vi "Ophir_ACQ.vi"(8 "error in (no error)":errorcluster, 10 "Background":dbl, 11 "Instruments in":refnum<class "Instruments.lvclass">) -> (0 "error out":errorcluster, 1 "Remeasure?":bool, 2 "Power,uW":dbl, 3 "Instruments out":refnum<class "Instruments.lvclass">, 5 "Back":dbl format="%0.2f")   [LabVIEW 2012, in "Instruments.lvclass"]
uses:
  Instruments.lvclass
  Instruments.lvclass/Instruments.ctl
  <vilib>/Analysis/NI_AALBase.lvlib
panel:
  out "Ophir_Param.Calibration Wl":dbl
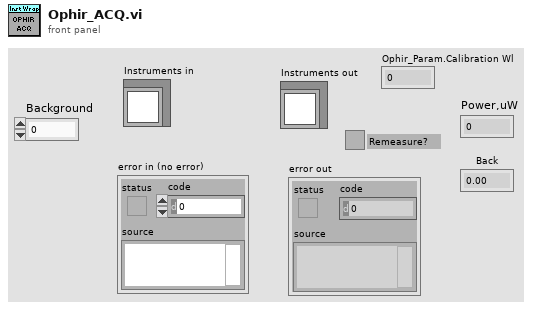
[diagram p1: front panel]
types:
  T1 = typedef "USB4000_Data.ctl" = cluster{"Wrapper Out":u32, "Number of Spectrometers":i32, "Wavelength":dbl[], "EL Spectrum":dbl[], "Int Time (usec)":i32, bool, "Background":dbl[]}
  T2 = cluster{"Keithley_Param":cluster{"Start Current,mA":dbl, "Stop Current,mA":dbl, "Voltage Compliance,V":dbl, "GPIB":string}, "USB4000_Param":cluster{"Integration Time":i32, "Wl min,nm":dbl, "Wl max,nm":dbl, "USB4000":T1}, "Ophir_Param":cluster{"VISA resource name":refnum<visa-resource-name>, "Calibration Wl":dbl}}
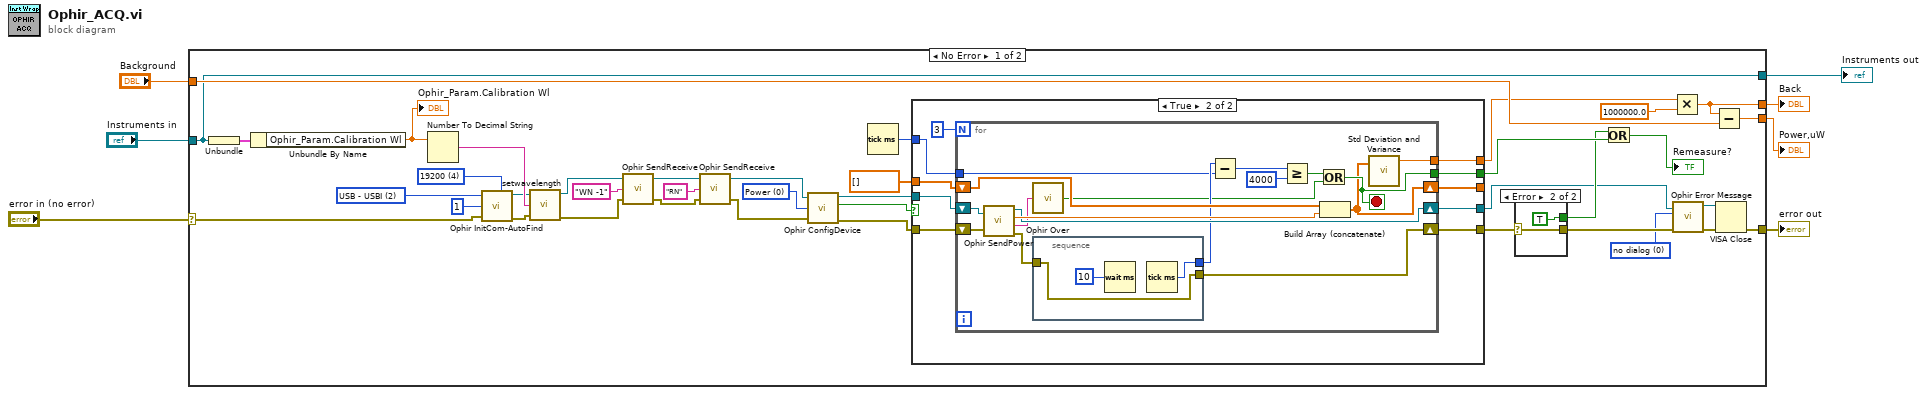
[diagram p0: block diagram]
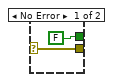
[diagram p2: hidden frame]
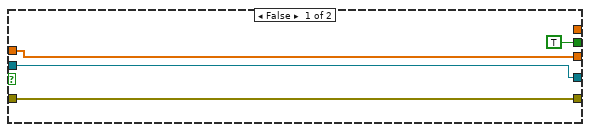
[diagram p3: hidden frame]
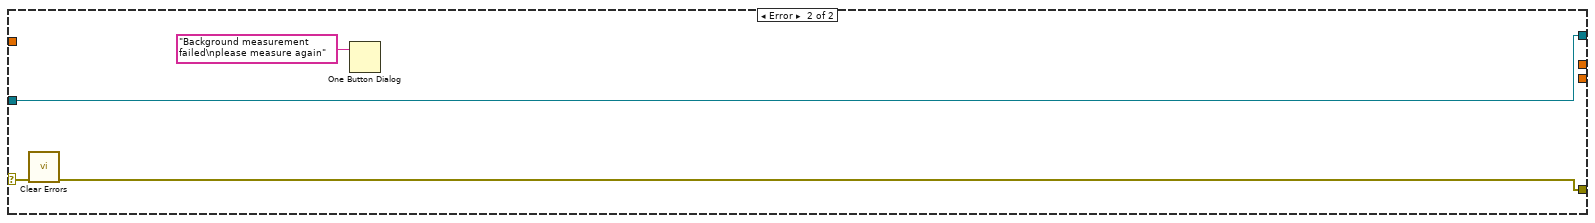
[diagram p4: hidden frame]
diagram:
  n1 = case shown="No Error" "error in (no error)" {
    selector: "error in (no error)" -> [w17 w86]
    tunnel: [w12 w85] -> w6
    tunnel: [w9 w88] -> w4
    tunnel: "Instruments in" -> [w9 w88]
    tunnel: "Background" -> [w24 _]
    tunnel: [w25 _] -> w2
    tunnel: [w23 _] -> w1
    frame No Error {
      w8 = 0 items=["no dialog", "OK message", "continue or stop message"] ("Type of Dialog (OK msg:1)")
      w18 = i16 4 items=["300", "1200", "4800", "9600", "19200", "38400"] ("Baud Rate (3:9600)")
      w20 = i16 2 items=["USB - Nova2", "USB - Vega", "USB - USBI", "RS232", "GPIB"] ("communication")
      w41 = u16 0 items=["Power", "Energy", "Frequency"] ("Measure Choice (0:Power)")
      n2 = Unbundle(w9) -> (w32:T2)
      n3 = Unbundle By Name(w32) -> ("Ophir_Param.Calibration Wl"=w21:dbl)
      "Ophir_Param.Calibration Wl" <- w21
      n4 = Number To Decimal String(number=w21) -> (decimal integer string=w33:string)  [unwired: 1 in]
      n5 = call "Ophir InitCom-AutoFind.vi"("Baud Rate (3:9600)"=w18, "communication"=w20, "Port Number (default 2)"=i16 1, "error in (no error)"=w17) -> ("Dup Visa Session"=w15:refnum<visa-resource-name>, "error out"=w16:errorcluster)  [unwired: 2 out]
      n6 = call "setwavelength.vi"("Dup Visa Session"=w15, "Set Wavelength"=w33, "error in (no error)"=w16) -> ("dup Visa Session"=w45:refnum<visa-resource-name>, "error out"=w44:errorcluster)  [unwired: 3 in]
      n7 = call "Ophir SendReceive.vi"("error in (no error)"=w44, "Command"="WN -1", "Visa Session"=w45) -> ("error out"=w29:errorcluster, "dup Visa Session"=w43:refnum<visa-resource-name>)  [unwired: 1 out]
      n8 = call "Ophir SendReceive.vi"("error in (no error)"=w29, "Command"="RN", "Visa Session"=w43) -> ("error out"=w39:errorcluster, "dup Visa Session"=w40:refnum<visa-resource-name>)  [unwired: 1 out]
      n9 = call "Ophir ConfigDevice.vi"("Visa Session"=w40, "Measure Choice (0:Power)"=w41, "error in (no error)"=w39) -> ("dup Visa Session"=w36:refnum<visa-resource-name>, "OK ?"=w38:bool, "error out"=w37:errorcluster)  [unwired: 1 out]
      n10 = Tick Count (ms)() -> (millisecond timer value=w30:u32)
      n11 = case shown="True" w38 {
        tunnel: w37 -> [w53 w62]
        tunnel: w36 -> [w54 w63]
        tunnel: dbl[] [] -> [w52 w64]
        tunnel: [w54 w61] -> w10
        tunnel: [w53 w60] -> w31
        tunnel: [w52 w59] -> _
        tunnel: w30 -> [_ w57]
        tunnel: [TRUE w56] -> w28
        tunnel: [_ w55] -> w22
        frame False {
        }
        frame True {
          n12 = for {
            N: 3 -> [_]
            shift-right: [w66] -> w59
            shift-left: w64 -> [w81]
            shift-right: [w77] -> w61
            shift-left: w63 -> [w79]
            shift-right: [w72] -> w60
            shift-left: w62 -> [w78]
            tunnel: w57 -> [w74]
            tunnel: [w67] -> w56
            tunnel: [w65] -> w55
            stop <- w67 stop-if-true
            n13 = call "Ophir SendPower.vi"("Visa Session"=w79, "error in (no error)"=w78) -> ("dup Visa Session"=w77:refnum<visa-resource-name>, "Value Number"=w80:dbl, "Value String"=w76:string, "error out"=w73:errorcluster)
            n14 = call "Ophir Over.vi"("Value String"=w76) -> ("Overrange"=w68:bool)
            n15 = stacked-sequence {
              tunnel: [w84] -> w75
              tunnel: w73 -> [w83]
              tunnel: [w83] -> w72
              frame #0 {
                n16 = Wait (ms)(milliseconds to wait=u32 10) -> ()  [unwired: 1 out]
                n17 = Tick Count (ms)() -> (millisecond timer value=w84:u32)
              }
            }
            n18 = Subtract(x=w75, y=w74) -> (x-y=w71:u32)
            n19 = Greater Or Equal?(x=w71, y=u32 4000) -> (x >= y?=w69:bool)
            n20 = Or(x=w69, y=w68) -> (x .or. y?=w67:bool)
            n21 = Build Array (concatenate)(w81, w80) -> (w66:dbl[])
            n22 = call <vilib>:"Std Deviation and Variance.vi"("X"=w66) -> ("mean"=w65:dbl)  [unwired: 1 in, 2 out]
          }
        }
      }
      n23 = case shown="Error" w31 {
        selector: w31 -> [w48 w49]
        tunnel: [w48 w49] -> w11
        tunnel: [FALSE ("x") TRUE ("x")] -> w26
        frame No Error {
        }
        frame Error {
        }
      }
      n24 = Or(x=w26, y=w28) -> (x .or. y?=→"Remeasure?":bool)
      n25 = Multiply(x=w22, y=1000000.0) -> (x*y=w25:dbl)
      n26 = call "Ophir Error Message.vi"("error in (no error)"=w11, "Type of Dialog (OK msg:1)"=w8, "Visa Session"=w10) -> ("error out"=w13:errorcluster, "dup Visa Session"=w14:refnum<visa-resource-name>)  [unwired: 1 in, 2 out]
      n27 = Subtract(x=w25, y=w24) -> (x-y=w23:dbl)
      n28 = VISA Close(VISA resource name=w14, error in (no error)=w13) -> (error out=w12:errorcluster)
    }
    frame Error {
      n29 = call <vilib>:"Clear Errors.vi"("error in (no error)"=w86) -> ("error out"=w85:errorcluster)  [unwired: 6 in]
      n30 = One Button Dialog(message="Background measurement failed\nplease measure again") -> ()  [unwired: 1 in, 1 out]
    }
  }
  "error out" <- w6
  "Instruments out" <- w4
  "Back" <- w2
  "Power,uW" <- w1
